vi "Hall_Sensor_FPGA.vi"(7 "Slope":enum16{"falling", "rising"}(ring), 8 "Hall Sensor":bool, 10 "Bounce time (uSec)":u32 caption="Bounce Time (uSec)") -> (0 "State Out":enum16{"Check Threshold", "Bounce Time"}(ring), 2 "Tach Period (uSec/pulse)":u32)   [LabVIEW 2019]
uses:
  <vilib>/rvi/Emulation/niFpgaGetClockAttributes.vi
  <vilib>/rvi/Emulation/niFpgaSctlEmulationGetInTimedLoop.vi
  <vilib>/rvi/Emulation/niFpgaEmulationReportErrorSimple.vi
  <vilib>/rvi/Emulation/niFpgaCriticalErrorInLSC.vi
  <vilib>/rvi/Arithmetic/AddSubMult/XNode/nirviSatArithmetic.xnode
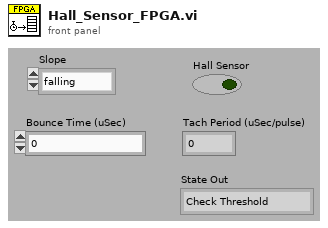
[diagram p1: front panel]
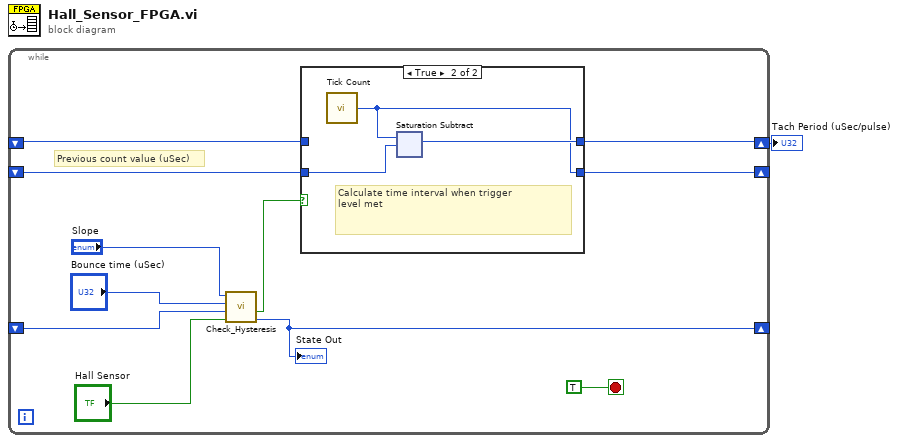
[diagram p0: block diagram]
diagram:
  n1 = while {
    shift-right: [w11] -> _
    shift-left: _ -> [w10]
    shift-right: [w3] -> _
    shift-left: _ -> [w2]
    shift-right: [w6] -> w1
    shift-left: _ -> [w9]
    stop <- TRUE stop-if-true
    # "Previous count value (uSec)"
    n2 = call "Check_Hysteresis.vi"("Hall Sensor"="Hall Sensor", "State In"=w2, "Bounce time (uSec)"="Bounce time (uSec)", "Slope"="Slope") -> ("State Out"=w3:enum16{"Check Threshold", "Bounce Time"}, "Event Ocurred?"=w8:bool)  [unwired: 3 in]
    "State Out" <- w3
    n3 = case shown="True" w8 {
      tunnel: w10 -> [w14 w17]
      tunnel: [w14 w15] -> w11
      tunnel: [w13 w16] -> w6
      tunnel: w9 -> [w13 _]
      frame False {
      }
      frame True {
        # "Calculate time interval when trigger\nlevel met"
        n4 = call "Tick Count"() -> ("Tick Count(uSec)"=w15:u32)
        n5 = xnode ("Saturation Subtract")("x"=w15, "y"=w17) -> ("x-y"=w16:u32)
      }
    }
  }
  "Tach Period (uSec/pulse)" <- w1
